vi "SCPI Initialize.vi"(7 "Serial Configuration":T1={"Baud Rate"=9600, "Parity"=0, "Data Bits"=8, "Stop Bits"=10, "Flow Control"=0} {"Flow Control" items=["None", "XON/XOFF", "RTS/CTS", "XON/XOFF & RTS/CTS", "DTR/DSR", "XON/XOFF & DTR/DSR"]; "Stop Bits" items=["1.0"=10, "1.5"=15, "2.0"=20]; "Data Bits" items=["7"=7, "8"=8]; "Parity" items=["None", "Odd", "Even", "Mark", "Space"]; "Baud Rate" items=["300"=300, "600"=600, "1200"=1200, "2400"=2400, "4800"=4800, "9600"=9600, "19200"=19200]}, 8 "error in (no error)":errorcluster, 10 "ID Query (True)":bool=TRUE, 11 "VISA resource name":refnum<visa-resource-name>) -> (0 "error out":errorcluster, 3 "VISA resource name out":refnum<visa-resource-name>)   [LabVIEW 2021, in "BK Precision 169XB.lvlib"]
doc: "Establishes communication with the instrument and optionally performs an instrument identification query and/or an instrument reset. It also places the instrument in a default state needed for other instrument driver operations. Therefore, call this VI before calling other instrument driver VIs for this instrument. Generally, you need to call the <b>Initialize</b> VI only once at the beginning of an application."
uses:
  BK Precision 169XB.lvlib
panel:
  # "(c) 2014 <Enter Company Name Here>.  ALL RIGHTS RESERVED."
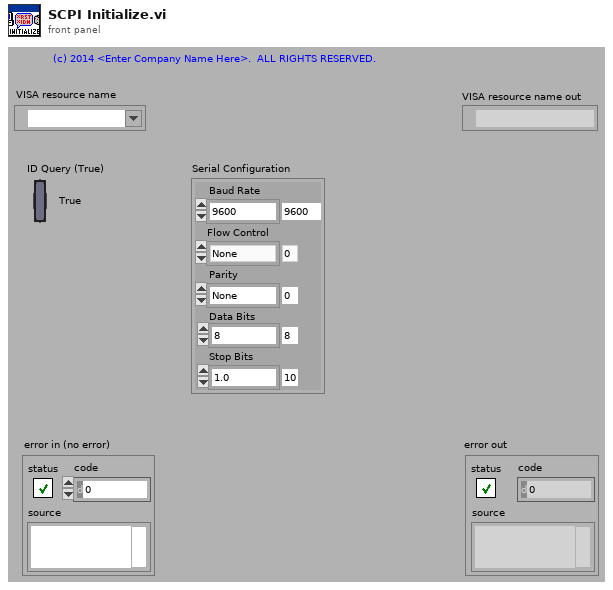
[diagram p1: front panel]
types:
  T1 = cluster{"Baud Rate":u32, "Parity":u16, "Data Bits":u16, "Stop Bits":u16, "Flow Control":u16}
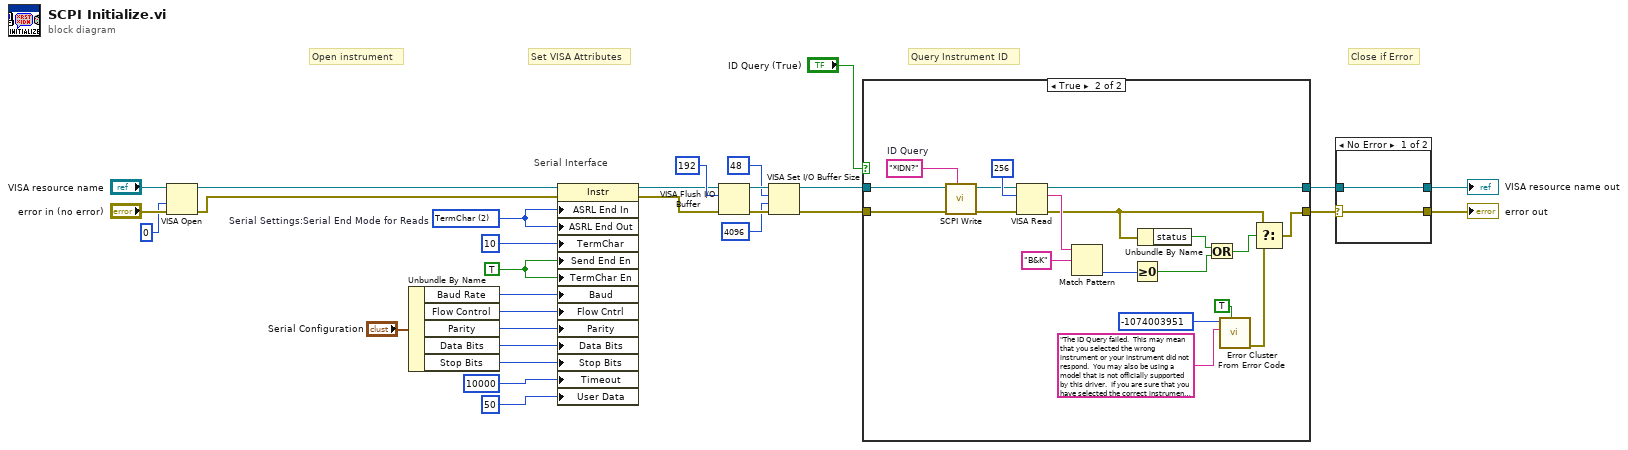
[diagram p0: block diagram]
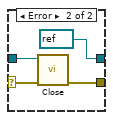
[diagram p2: hidden frame]
diagram:
  w6 = TRUE ("Message Based Settings:Termination Character Enable")
  w9 = u16 2 items=["None", "LastBit", "TermChar"]  # Serial Settings:Serial End Mode for Reads
  # "Serial Interface"
  # "Set VISA Attributes"
  # "Close if Error"
  # "Query Instrument ID"
  # "Open instrument"
  n1 = VISA Open(access mode=u32 0, error in (no error)="error in (no error)", VISA resource name="VISA resource name") -> (VISA resource name=w26:refnum<visa-resource-name>, error out=w25:errorcluster)  [unwired: 2 in]
  n2 = Unbundle By Name("Serial Configuration") -> ("Baud Rate"=w7:u32, "Flow Control"=w13:u16, "Parity"=w12:u16, "Data Bits"=w11:u16, "Stop Bits"=w8:u16)
  n3 = property class="Instr"(reference=w26, error in=w25, "ASRL End In"=w9, "ASRL End Out"=w9, "TermChar"=u8 10 ("Message Based Settings:Termination Character"), "Send End En"=w6, "TermChar En"=w6, "Baud"=w7, "Flow Cntrl"=w13, "Parity"=w12, "Data Bits"=w11, "Stop Bits"=w8, "Timeout"=u32 10000 ("General Settings:Timeout Value"), "User Data"=u32 50 ("General Settings:User Data")) -> (reference out=w15:refnum<visa-resource-name>, error out=w14:errorcluster)
  n4 = VISA Flush I/O Buffer(VISA resource name=w15, mask (16)=u16 192, error in (no error)=w14) -> (VISA resource name out=w22:refnum<visa-resource-name>, error out=w21:errorcluster)
  n5 = VISA Set I/O Buffer Size(VISA resource name=w22, mask (16)=u16 48, size (4096)=u32 4096 ("size (0)"), error in (no error)=w21) -> (VISA resource name out=w17:refnum<visa-resource-name>, error out=w16:errorcluster)
  n6 = case shown="True" "ID Query (True)" {
    tunnel: [w31 w51] -> w2
    tunnel: [w32 w50] -> w1
    tunnel: w17 -> [w32 w33]
    tunnel: w16 -> [w31 w36]
    frame False {
    }
    frame True {
      w34 = "*IDN?"  # ID Query
      n7 = call "SCPI Write.vi"("Input String"=w34, "error in (no error)"=w36, "VISA resource name"=w33) -> ("error out"=w37:errorcluster, "VISA resource name out"=w35:refnum<visa-resource-name>)  [unwired: 7 in]
      n8 = VISA Read(VISA resource name=w35, byte count=u32 256, error in (no error)=w37) -> (VISA resource name out=w50:refnum<visa-resource-name>, read buffer=w49:string, error out=w41:errorcluster)  [unwired: 1 out]
      n9 = Match Pattern(string=w49, regular expression="B&K") -> (offset past match=w42:i32)  [unwired: 1 in, 3 out]
      n10 = Greater Or Equal To 0?(x=w42) -> (x >= 0?=w39:bool)
      n11 = Unbundle By Name(w41) -> ("status"=w40:bool)
      n12 = Or(x=w40, y=w39) -> (x .or. y?=w38:bool)
      n13 = call <vilib>:"Error Cluster From Error Code.vi"("show call chain? (False)"=TRUE, "error message (\"\")"="The ID Query failed.  This may mean that you selected the wrong instrument or your instrument did not respond.  You may also be using a model that is not officially supported by this driver.  If you are sure that you have selected the correct instrument and it is responding, try disabling the ID Query." ("Source (VI Name)"), "error code (0)"=-1074003951 ("Code")) -> ("error out"=w46:errorcluster)  [unwired: 6 in]
      n14 = Select(t=w41, s=w38, f=w46) -> (s? t:f=w51:errorcluster)
    }
  }
  n15 = case shown="No Error" w2 {
    selector: w2 -> [w53 w55]
    tunnel: [w52 refnum<visa-resource-name> refnum ("VISA resource name out")] -> w24
    tunnel: [w53 w56] -> w23
    tunnel: w1 -> [w52 w54]
    frame No Error {
    }
    frame Error {
      n16 = call "Close.vi"("error in (no error)"=w55, "VISA resource name"=w54) -> ("error out"=w56:errorcluster)  [unwired: 9 in]
    }
  }
  "VISA resource name out" <- w24
  "error out" <- w23
